vi "Write.vi"(8 "error in (no error)":errorcluster, 9 "timeout ms (25000)":i32, 10 "Bytes to write":u8[](array[numeric]), 11 "Socket in":refnum<class "Socket.lvclass">) -> (0 "error out":errorcluster, 2 "bytes written":i32, 3 "Socket out":refnum<class "Socket.lvclass">)   [LabVIEW 2013, in "Sockets.lvlib" / "Socket.lvclass"]
doc: "Writes data to the socket."
uses:
  Socket.lvclass
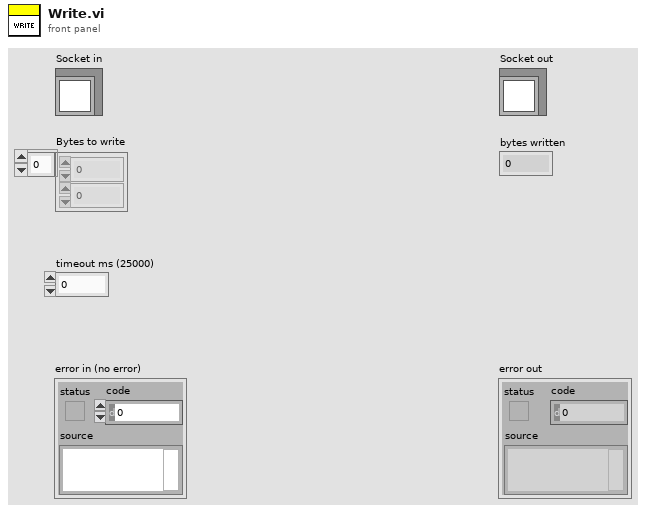
[diagram p1: front panel]
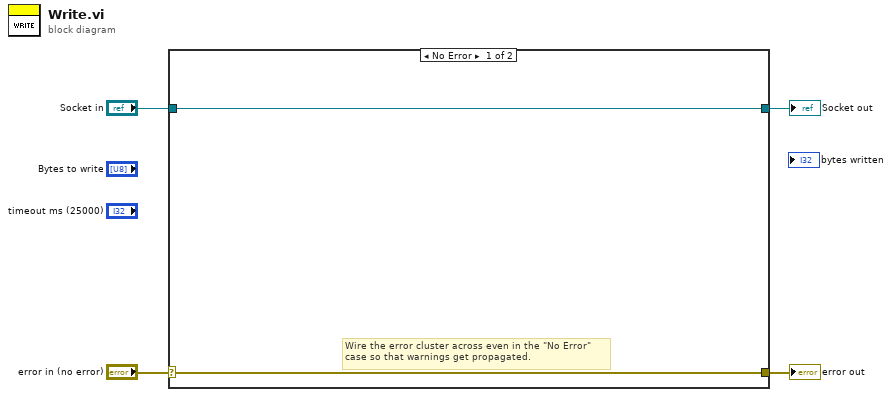
[diagram p0: block diagram]
diagram:
  n1 = case shown="No Error" "error in (no error)" {
    selector: "error in (no error)" -> [w5 w8]
    tunnel: [w5 w8] -> w3
    tunnel: [w6 w7] -> w1
    tunnel: "Socket in" -> [w6 w7]
    frame No Error {
      # "Wire the error cluster across even in the \"No Error\"\ncase so that warnings get propagated."
    }
    frame Error {
    }
  }
  "error out" <- w3
  "Socket out" <- w1
